vi "motorReverse.vi"() -> ()   [LabVIEW 2017]
panel:
  in  "motorsRun":bool
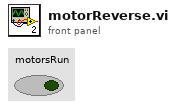
[diagram p1: front panel]
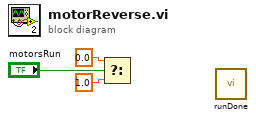
[diagram p0: block diagram]
diagram:
  n1 = Select(t=0.0, s="motorsRun", f=1.0) -> ()  [unwired: 1 out]
  n2 = call "runDone.vi"() -> ()  [unwired: 11 in, 1 out]
